vi "Read Current Command Code.vi"(8 "error in (no error)":errorcluster, 11 "AK RS232 in":refnum<class "AK RS-xxx.lvclass">) -> (0 "error out":errorcluster, 2 "Current Command Code":string, 3 "AK RS232 out":refnum<class "AK RS-xxx.lvclass">)   [LabVIEW 2013, in "Protocol Classes.lvlib" / "AK RS-xxx.lvclass"]
uses:
  AK RS-xxx.lvclass
  AK RS-xxx.lvclass/AK RS-xxx.ctl
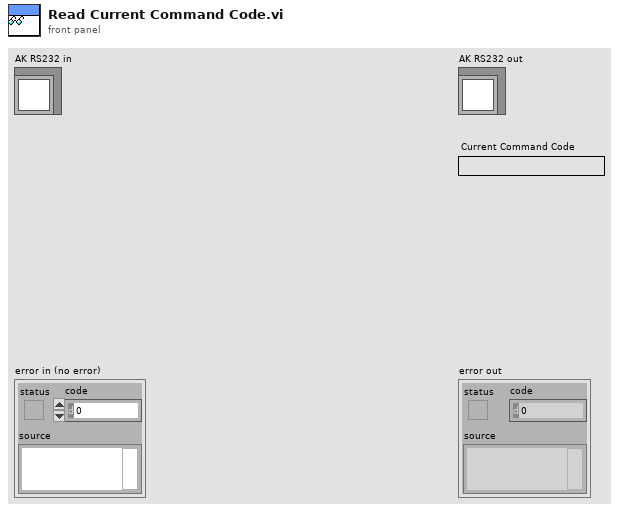
[diagram p1: front panel]
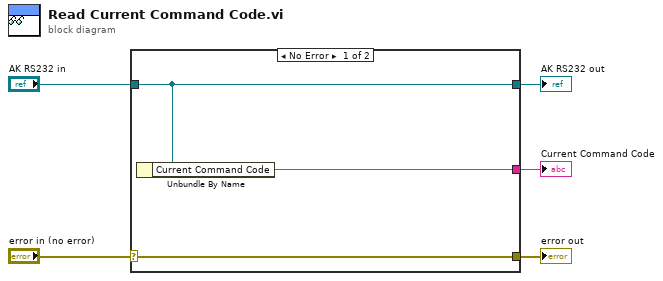
[diagram p0: block diagram]
diagram:
  n1 = case shown="No Error" "error in (no error)" {
    selector: "error in (no error)" -> [w8 w9]
    tunnel: [w8 w9] -> w4
    tunnel: [w7 w10] -> w2
    tunnel: "AK RS232 in" -> [w7 w10]
    tunnel: [w6 _] -> w1
    frame No Error {
      n2 = Unbundle By Name(w7) -> ("Current Command Code"=w6:string)
    }
    frame Error {
    }
  }
  "error out" <- w4
  "AK RS232 out" <- w2
  "Current Command Code" <- w1
